vi "Memory Manager Post-Build.vi"   [LabVIEW 2017]
uses:
  Build Automation.lvlib
types:
  T1 = cluster{"Status Message":refnum<data-value>, "Progress":refnum<data-value>, "Stop":refnum<data-value>}
  T2 = enum16{"Share clones between instances", "Preallocate clone for each instance"}
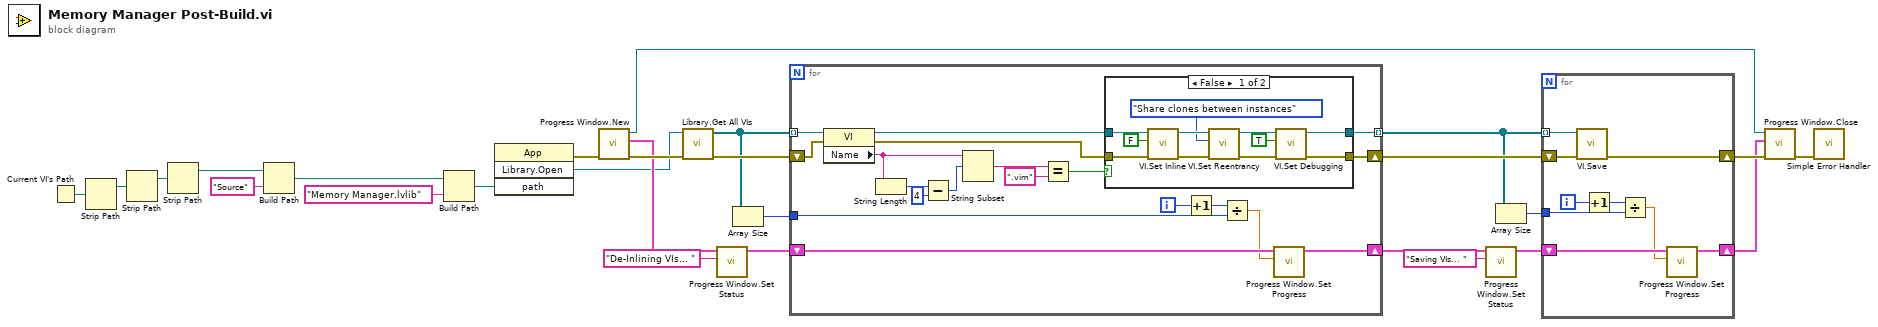
[diagram p0: block diagram]
diagram:
  n1 = Current VI's Path() -> (path=w26:path)
  n2 = Strip Path(path=w26) -> (stripped path=w25:path)  [unwired: 1 out]
  n3 = Strip Path(path=w25) -> (stripped path=w24:path)  [unwired: 1 out]
  n4 = Strip Path(path=w24) -> (stripped path=w23:path)  [unwired: 1 out]
  n5 = Build Path(base path=w23, name or relative path="Source") -> (appended path=w22:path)
  n6 = Build Path(base path=w22, name or relative path="Memory Manager.lvlib" ("library name")) -> (appended path=w20:path)
  n7 = invoke class="App" method="Library.Open"("path"=w20) -> (error out=w18:errorcluster, "Open Library"=w6:refnum<vi>)  [unwired: 3 in, 2 out]
  n8 = call "Progress Window.New.vi"("error in (no error)"=w18) -> ("error out"=w8:errorcluster, "DVRs"=w7:T1, "VI refnum"=w12:refnum<vi>)  [unwired: 8 in]
  n9 = call "Library.Get All VIs.vi"("error in (no error)"=w8, "library ref"=w6) -> ("error out"=w19:errorcluster, "vi refs"=w16:refnum<vi>[])  [unwired: 8 in]
  n10 = call "Progress Window.Set Status.vi"("Status Message"="De-Inlining VIs... " ("data value"), "DVRs in"=w7) -> ("DVRs out"=w14:T1)  [unwired: 8 in, 1 out]
  n11 = Array Size(array=w16) -> (size(s)=w15:i32)
  n12 = for {
    tunnel: w16 -> [w32] mode=indexing
    shift-right: [w39] -> w11
    shift-left: w19 -> [w31]
    tunnel: w15 -> [w44]
    shift-right: [w41] -> w10
    shift-left: w14 -> [w43]
    tunnel: [w40] -> w4 mode=indexing
    i -> [w46]
    n13 = property class="VI"(reference=w32, error in=w31) -> (reference out=w30:refnum<vi>, error out=w29:errorcluster, "Name"=w38:string)
    n14 = String Length(string=w38) -> (length=w37:i32)
    n15 = Subtract(x=w37, y=4) -> (x-y=w33:i32)
    n16 = String Subset(string=w38, offset (0)=w33) -> (substring=w35:string)  [unwired: 1 in]
    n17 = Equal?(x=w35, y=".vim") -> (x = y?=w28:bool)
    n18 = case shown="False" w28 {
      tunnel: [w50 w59] -> w40
      tunnel: [w49 w58] -> w39
      tunnel: w30 -> [w48 w59]
      tunnel: w29 -> [w47 w58]
      frame False {
        n19 = call "VI.Set Inline.vi"("error in (no error)"=w47, "Inline VI"=FALSE, "vi ref in"=w48) -> ("error out"=w54:errorcluster, "vi ref out"=w55:refnum<vi>)  [unwired: 7 in]
        n20 = call "VI.Set Reentrancy.vi"("error in (no error)"=w54, "Reentrancy Type"=T2."Share clones between instances", "vi ref in"=w55) -> ("error out"=w51:errorcluster, "vi ref out"=w52:refnum<vi>)  [unwired: 7 in]
        n21 = call "VI.Set Debugging.vi"("error in (no error)"=w51, "Allow Debugging"=TRUE, "vi ref in"=w52) -> ("error out"=w49:errorcluster, "vi ref out"=w50:refnum<vi>)  [unwired: 7 in]
      }
      frame True {
      }
    }
    n22 = Increment(x=w46) -> (x+1=w45:i32)
    n23 = Divide(x=w45, y=w44) -> (x/y=w42:dbl)
    n24 = call "Progress Window.Set Progress.vi"("Progress"=w42, "DVRs in"=w43) -> ("DVRs out"=w41:T1)  [unwired: 8 in, 1 out]
  }
  n25 = call "Progress Window.Set Status.vi"("Status Message"="Saving VIs... ", "DVRs in"=w10) -> ("DVRs out"=w5:T1)  [unwired: 8 in, 1 out]
  n26 = Array Size(array=w4) -> (size(s)=w3:i32)
  n27 = for {
    shift-right: [w66] -> w2
    shift-left: w11 -> [w68]
    tunnel: w4 -> [w67] mode=indexing
    shift-right: [w60] -> w1
    shift-left: w5 -> [w62]
    tunnel: w3 -> [w64]
    i -> [w63]
    n28 = call "VI.Save.vi"("error in (no error)"=w68, "vi ref in"=w67) -> ("error out"=w66:errorcluster)  [unwired: 8 in, 1 out]
    n29 = Increment(x=w63) -> (x+1=w65:i32)
    n30 = Divide(x=w65, y=w64) -> (x/y=w61:dbl)
    n31 = call "Progress Window.Set Progress.vi"("Progress"=w61, "DVRs in"=w62) -> ("DVRs out"=w60:T1)  [unwired: 8 in, 1 out]
  }
  n32 = call "Progress Window.Close.vi"("error in (no error)"=w2, "DVRs in"=w1, "VI refnum"=w12) -> ("error out"=w13:errorcluster)  [unwired: 8 in]
  n33 = call <vilib>:"Simple Error Handler.vi"("error in (no error)"=w13) -> ()  [unwired: 4 in, 5 out]
